vi "PC Data Clear.vi"(8 "errorIN":errorcluster caption="Error", 9 "usegates?":bool caption="Use Gates", 11 "Photon Counter SR400 in":refnum<class "Photon Counter.lvclass">) -> (0 "errorOUT":errorcluster caption="Error", 3 "Photon Counter SR400 out":refnum<class "Photon Counter.lvclass">)   [LabVIEW 2017, in "Photon Counter.lvclass"]
uses:
  Photon Counter.lvclass
  Photon Counter.lvclass/Photon Counter.ctl
  SR400/SR400.lvlib
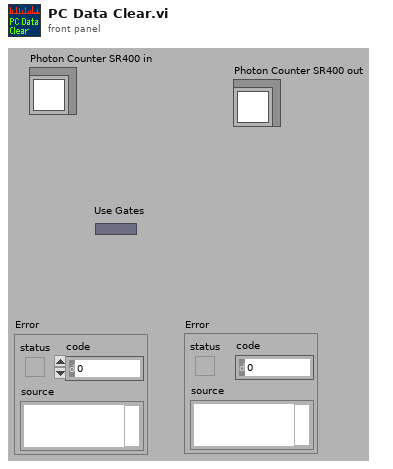
[diagram p1: front panel]
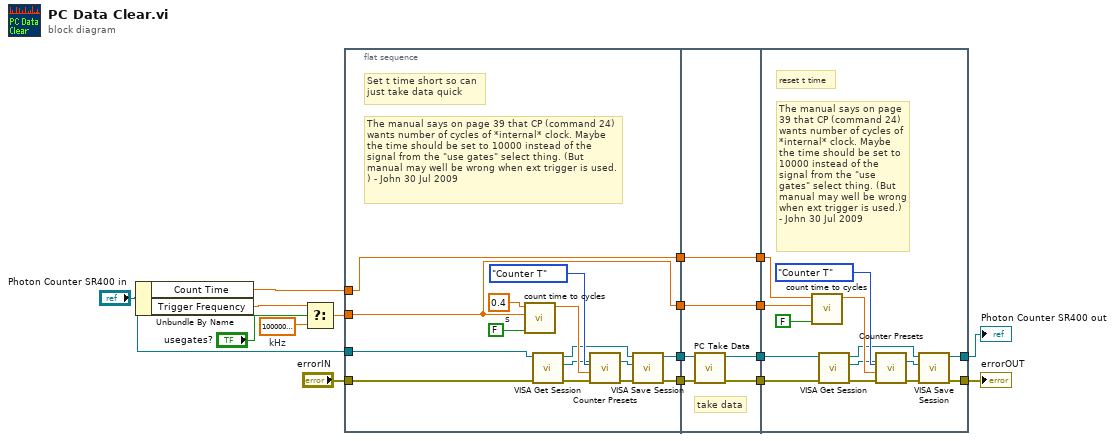
[diagram p0: block diagram]
diagram:
  w13 = dbl[unit] 10000000.0  # kHz
  n1 = Unbundle By Name("Photon Counter SR400 in") -> ("Count Time"=w3:dbl[unit], "Trigger Frequency"=w2:dbl[unit])
  n2 = Select(t=w2, s="usegates?", f=w13) -> (s? t:f=w14:dbl[unit])
  n3 = flat-sequence {
    tunnel: "errorIN" -> [w22]
    tunnel: w14 -> [w32]
    tunnel: [w32] -> w12
    tunnel: w3 -> [w27]
    tunnel: [w27] -> w11
    tunnel: "Photon Counter SR400 in" -> [w23]
    tunnel: [w19] -> w5
    tunnel: [w18] -> w1
    tunnel: [w36] -> w10
    tunnel: w12 -> [w38]
    tunnel: [w38] -> w9
    tunnel: w11 -> [w37]
    tunnel: [w37] -> w8
    tunnel: [w35] -> w7
    tunnel: w5 -> [w34]
    tunnel: w1 -> [w33]
    tunnel: [w39] -> w17
    tunnel: w10 -> [w42]
    tunnel: w9 -> [w50]
    tunnel: w8 -> [w52]
    tunnel: w7 -> [w41]
    tunnel: [w40] -> w6
    frame #0 {
      w31 = dbl[unit] 0.4  # s
      # "The manual says on page 39 that CP (command 24) wants number of cycles of *internal* clock. Maybe the time should be set to 10000 instead of the signal from the \"use gates\" select thing. (But manual may well be wrong when ext trigger is used.) - John 30 Jul 2009"
      # "Set t time short so can\njust take data quick"
      n4 = call "count time to cycles.vi"("dispmsg?"=FALSE, "Trigger Freq"=w32, "Count Time Set"=w31) -> ("Number of triggers"=w28:dbl)  [unwired: 4 out]
      n5 = call-dynamic "VISA Get Session.vi"("error in (no error)"=w22, "Instrument.lvclass in"=w23) -> ("error out"=w21:errorcluster, "VISA Resource Name"=w25:refnum<visa-resource-name>, "Instrument.lvclass out"=w24:refnum<class "Photon Counter.lvclass">)  [unwired: 7 out]
      n6 = call "Counter Presets.vi"("error in (no error)"=w21, "Number of triggers"=w28, "Counter (Def: T)"=enum16{"Invalid", "Counter B", "Counter T"}."Counter T" ("i (0) 2"), "VISA resource name"=w25) -> ("error out"=w20:errorcluster, "VISA resource name out"=w26:refnum<visa-resource-name>)  [unwired: 6 out]
      n7 = call-dynamic "VISA Save Session.vi"("error in (no error)"=w20, "VISA Resource Name"=w26, "Instrument.lvclass in"=w24) -> ("error out"=w18:errorcluster, "Instrument.lvclass out"=w19:refnum<class "Photon Counter.lvclass">)  [unwired: 7 out]
    }
    frame #1 {
      # "take data"
      n8 = call "PC Take Data.vi"("error in (no error)"=w33, "Photon Counter SR400 in"=w34) -> ("error out"=w36:errorcluster, "Photon Counter SR400 out"=w35:refnum<class "Photon Counter.lvclass">)  [unwired: 4 in, 4 out]
    }
    frame #2 {
      # "The manual says on page 39 that CP (command 24) wants number of cycles of *internal* clock. Maybe the time should be set to 10000 instead of the signal from the \"use gates\" select thing. (But manual may well be wrong when ext trigger is used.) - John 30 Jul 2009"
      # "reset t time"
      n9 = call "count time to cycles.vi"("dispmsg?"=FALSE, "Trigger Freq"=w50, "Count Time Set"=w52) -> ("Number of triggers"=w49:dbl)  [unwired: 4 out]
      n10 = call-dynamic "VISA Get Session.vi"("error in (no error)"=w42, "Instrument.lvclass in"=w41) -> ("error out"=w43:errorcluster, "VISA Resource Name"=w46:refnum<visa-resource-name>, "Instrument.lvclass out"=w47:refnum<class "Photon Counter.lvclass">)  [unwired: 7 out]
      n11 = call "Counter Presets.vi"("error in (no error)"=w43, "Number of triggers"=w49, "Counter (Def: T)"=enum16{"Invalid", "Counter B", "Counter T"}."Counter T" ("i (0) 2"), "VISA resource name"=w46) -> ("error out"=w44:errorcluster, "VISA resource name out"=w45:refnum<visa-resource-name>)  [unwired: 1 in, 5 out]
      n12 = call-dynamic "VISA Save Session.vi"("error in (no error)"=w44, "VISA Resource Name"=w45, "Instrument.lvclass in"=w47) -> ("error out"=w39:errorcluster, "Instrument.lvclass out"=w40:refnum<class "Photon Counter.lvclass">)  [unwired: 7 out]
    }
  }
  "errorOUT" <- w17
  "Photon Counter SR400 out" <- w6
